vi "testing.vi"() -> ()   [LabVIEW 2017]
panel:
  in  "stop":bool
  out "Fahrenheit":dbl
  out "Thermometer":dbl(slide) scale=0.0..212.0
  out "Celcius":dbl
  in  "?":dbl(slide) scale=0.0..100.0
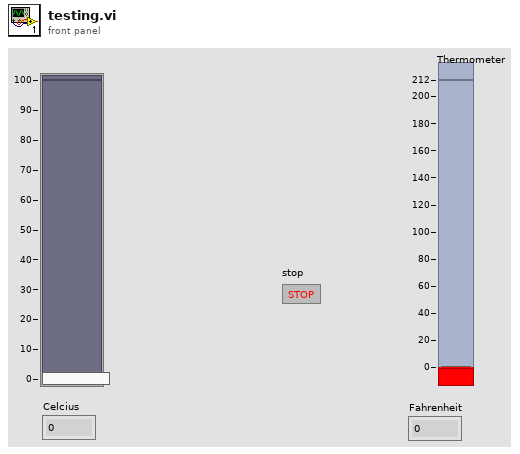
[diagram p1: front panel]
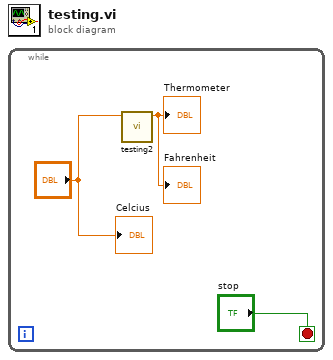
[diagram p0: block diagram]
diagram:
  n1 = while {
    stop <- "stop" stop-if-true
    n2 = call "testing2.vi"("Numeric in"="?") -> ("Numeric out"=→"Thermometer" →"Fahrenheit":dbl)  [unwired: 10 in]
    "Celcius" <- "?"
  }
